vi "LinearScale.vi"(9 "Offset":dbl, 10 "Slope":dbl, 11 "Voltage":dbl) -> (2 "ScaledOut":dbl, 3 "Vout":dbl)   [LabVIEW 2018]
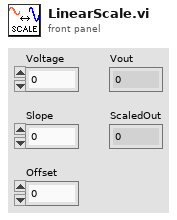
[diagram p1: front panel]
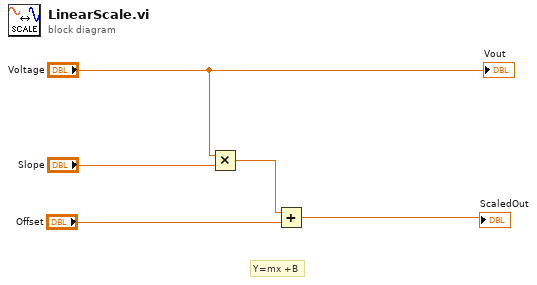
[diagram p0: block diagram]
diagram:
  # "Y=mx +B"
  n1 = Multiply(x="Voltage", y="Slope") -> (x*y=w1:dbl)
  n2 = Add(x=w1, y="Offset") -> (x+y=→"ScaledOut":dbl)
  "Vout" <- "Voltage"
